vi "prueba2_21311001_grethelcruz.vi"() -> ()   [LabVIEW 2013]
panel:
  out "mayor":dbl
  out "Menor":dbl
  out "Temperatura80":dbl
  out "Promedio":dbl
  out "Velocidad":i32(knob) scale=0.0..220.0
  # "Necesitamos generar 10 velocidades. \nal final de las 10 pruebas presentar :\n-Promedio de las velocidades mayores a 120\n-Velocidad Mayor y menor \n-Cuantas veces la temperatura fue mayor a 80"
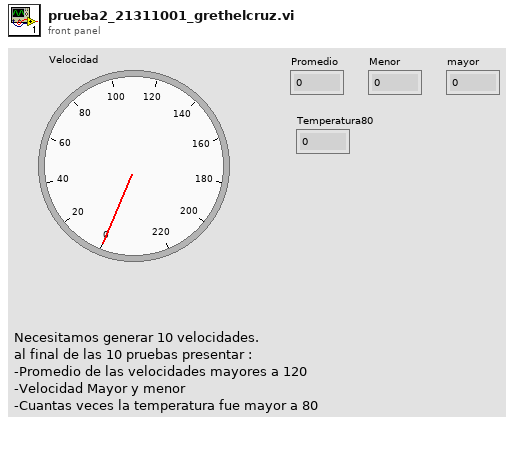
[diagram p1: front panel]
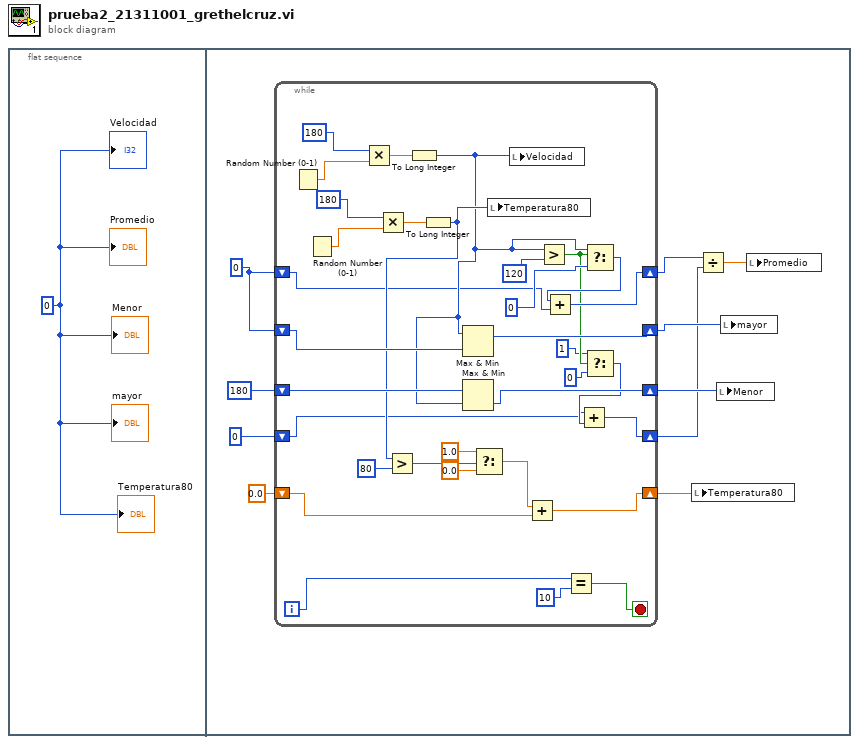
[diagram p0: block diagram]
diagram:
  n1 = flat-sequence {
    frame #0 {
      w1 = 0
      "Velocidad" <- w1
      "Promedio" <- w1
      "Menor" <- w1
      "mayor" <- w1
      "Temperatura80" <- w1
    }
    frame #1 {
      w9 = 0
      n2 = while {
        shift-right: [w18] -> w10
        shift-left: w9 -> [w19]
        shift-right: [w34] -> w7
        shift-left: w9 -> [w33]
        shift-right: [w31] -> w6
        shift-left: 180 -> [w32]
        shift-right: [w23] -> w4
        shift-left: 0.0 ("f") -> [w24]
        shift-right: [w12] -> w3
        shift-left: 0 -> [w13]
        i -> [w37]
        stop <- w38 stop-if-true
        n3 = Random Number (0-1)() -> (number: 0 to 1=w43:dbl)
        n4 = Random Number (0-1)() -> (number: 0 to 1=w40:dbl)
        n5 = Multiply(x=180, y=w43) -> (x*y=w42:dbl)
        n6 = Multiply(x=180, y=w40) -> (x*y=w41:dbl)
        n7 = To Long Integer(number=w42) -> (32bit integer=w22:i32)
        n8 = To Long Integer(number=w41) -> (32bit integer=w30:i32)
        n9 = Greater?(x=w30, y=80) -> (0:w28:bool)
        n10 = Max & Min(x=w22, y=w33) -> (max(x,y)=w34:i32)  [unwired: 1 out]
        n11 = Max & Min(x=w32, y=w22) -> (min(x,y)=w31:i32)  [unwired: 1 out]
        n12 = Select(t=1.0, s=w28, f=0.0) -> (s? t:f=w25:dbl)
        n13 = local write "Temperatura80"(w30) -> ()
        n14 = local write "Velocidad"(w22) -> ()
        n15 = Add(x=w25, y=w24) -> (x+y=w23:dbl)
        n16 = Greater?(x=w22, y=120) -> (0:w17:bool)
        n17 = Equal?(x=w37, y=10) -> (x = y?=w38:bool)
        n18 = Select(t=w22, s=w17, f=0) -> (s? t:f=w21:i32)
        n19 = Add(x=w21, y=w19) -> (x+y=w18:i32)
        n20 = Select(t=1, s=w17, f=0) -> (s? t:f=w14:i32)
        n21 = Add(x=w13, y=w14) -> (x+y=w12:i32)
      }
      n22 = local write "Temperatura80"(w4) -> ()
      n23 = Divide(x=w10, y=w3) -> (x/y=w11:dbl)
      n24 = local write "Menor"(w6) -> ()
      n25 = local write "mayor"(w7) -> ()
      n26 = local write "Promedio"(w11) -> ()
    }
  }
